vi "ShooterTEST.vi"(5 "WinchCaseIn":dbl, 8 "OutGearPos":dbl=2.1, 9 "InGearPos":dbl=1.5, 10 "Pot":dbl, 11 "Fire":bool) -> (0 "There?":bool, 1 "WinchCase":i32, 3 "Power":dbl)   [LabVIEW 2013]
panel:
  out "Index":i32
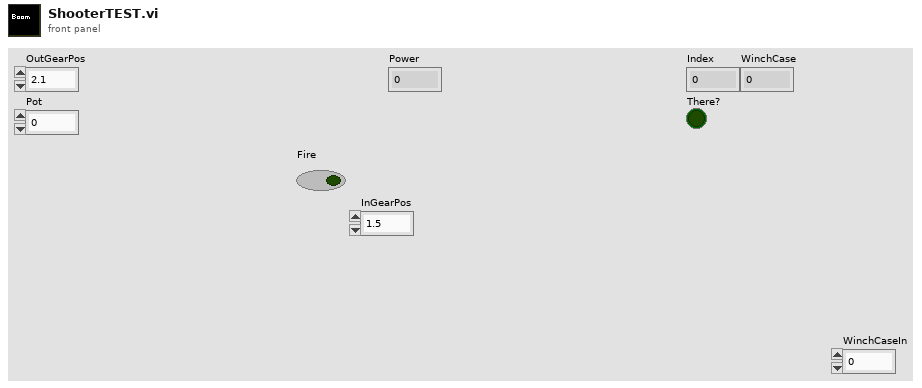
[diagram p1: front panel]
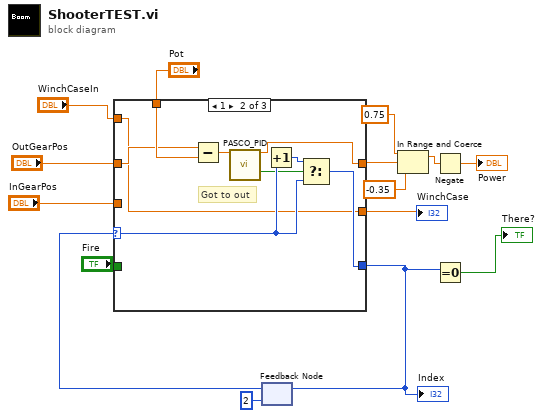
[diagram p0: block diagram]
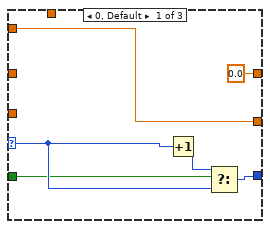
[diagram p2: hidden frame]
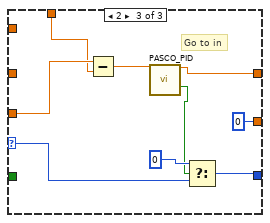
[diagram p3: hidden frame]
diagram:
  n1 = feedback #1(2 ("Numeric")) -> (w13:i32)
  n2 = case shown="1" w13 {
    selector: w13 -> [w19 w28 w37]
    tunnel: [0.0 ("Output") w27 w36] -> w6
    tunnel: "Fire" -> [w18 _ _]
    tunnel: [w21 w30 w39] -> w10
    tunnel: "OutGearPos" -> [_ w23 _]
    tunnel: "InGearPos" -> [_ _ w34]
    tunnel: "Pot" -> [_ w24 w33]
    tunnel: [w16 w22 0 ("WinchCase")] -> w7
    tunnel: "WinchCaseIn" -> [w16 w22 _]
    frame 0, Default {
      n3 = Increment(x=w19) -> (x+1=w20:i32)
      n4 = Select(t=w20, s=w18, f=w19) -> (s? t:f=w21:i32)
    }
    frame 1 {
      # "Got to out"
      n5 = Subtract(x=w23, y=w24) -> (x-y=w25:dbl)
      n6 = call "PASCO_PID.vi"("Delta"=w25) -> ("Output"=w27:dbl, "IsThere"=w26:bool)  [unwired: 13 in]
      n7 = Increment(x=w28) -> (x+1=w29:i32)
      n8 = Select(t=w29, s=w26, f=w28) -> (s? t:f=w30:i32)
    }
    frame 2 {
      # "Go to in"
      n9 = Subtract(x=w34, y=w33) -> (x-y=w32:dbl)
      n10 = call "PASCO_PID.vi"("Delta"=w32) -> ("Output"=w36:dbl, "IsThere"=w35:bool)  [unwired: 13 in]
      n11 = Select(t=0, s=w35, f=w37) -> (s? t:f=w39:i32)
    }
  }
  "Index" <- w10
  "WinchCase" <- w7
  n12 = feedback-in #1(w10) -> ()
  n13 = In Range and Coerce(upper limit=0.75, x=w6, lower limit=-0.35) -> (coerced(x)=w3:dbl)  [unwired: 1 out]
  n14 = Negate(x=w3) -> (-x=→"Power":dbl)
  n15 = Equal To 0?(x=w10) -> (x = 0?=→"There?":bool)
